vi "GV_YscaleAddText.vi"(4 "Color":u32(colorbox), 6 "X-position":i16, 7 "Tagname":string, 8 "Scale top":i16, 9 "Plot bottom":i16, 11 "2D Picture IN":picture) -> (3 "2D Picture OUT":picture)   [LabVIEW 2020, in "Sgraph_lib_V1.lvlib" / "Gviewer.lvclass"]
doc: "Andre Koelewijn, 25 July 2021\n\nThis vi will add a tagname to the Y scale."
uses:
  Gviewer.lvclass
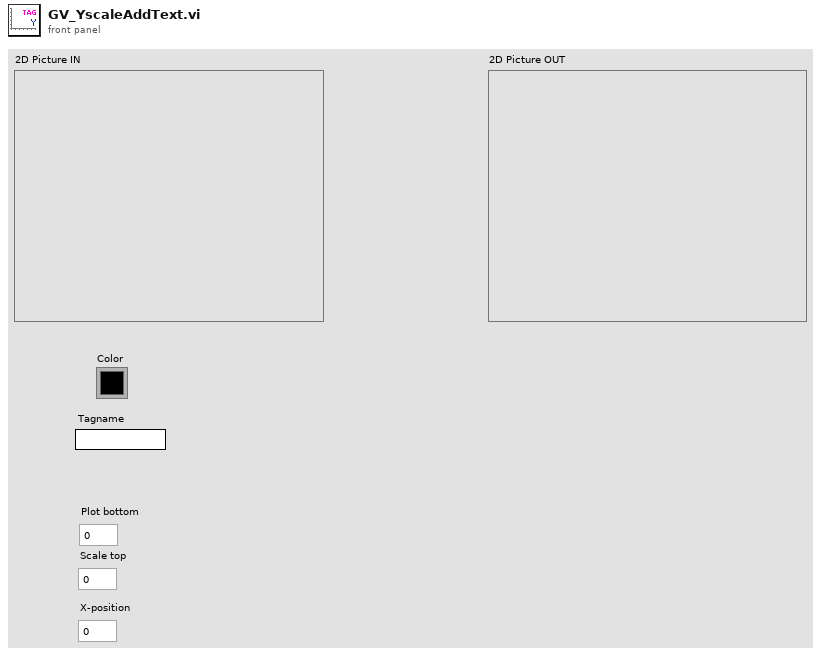
[diagram p1: front panel]
types:
  T1 = cluster{"horizontal":enum16{"left", "center", "right"}, "vertical":enum16{"top", "center", "bottom"}}
  T2 = cluster{"left":i16, "top":i16, "right":i16, "bottom":i16}
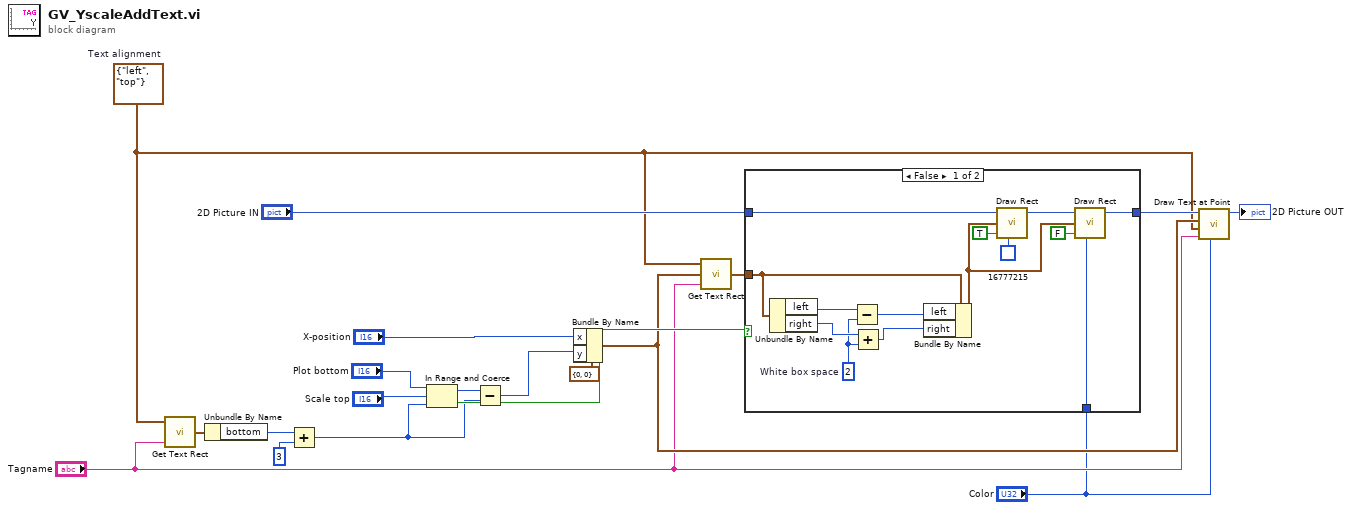
[diagram p0: block diagram]
diagram:
  w5 = T1 {"horizontal"=enum."left", "vertical"=enum."top"}  # Text alignment
  n1 = call <vilib>:"Get Text Rect.vi"("alignment(left, top)"=w5, "text"="Tagname") -> ("rect"=w13:T2)  [unwired: 7 in]
  n2 = Unbundle By Name(w13) -> ("bottom"=w12:i16)
  n3 = Add(x=w12, y=i16 3) -> (x+y=w2:i16)
  n4 = In Range and Coerce(upper limit="Plot bottom", x="Scale top", lower limit=w2) -> (coerced(x)=w10:i16, In Range?=w18:bool)
  n5 = Subtract(x=w10, y=w2) -> (x-y=w8:i16)
  n6 = Bundle By Name(cluster=cluster{"x":i16, "y":i16} {"x"=0, "y"=0} ("origin"), "x"="X-position", "y"=w8) -> (w7:cluster{"x":i16, "y":i16})
  n7 = call <vilib>:"Get Text Rect.vi"("alignment(left, top)"=w5, "origin(0,0)"=w7, "text"="Tagname") -> ("rect"=w4:T2)  [unwired: 6 in]
  n8 = case shown="False" w18 {
    tunnel: "2D Picture IN" -> [w33 w34]
    tunnel: [w31 w34] -> w16
    tunnel: w4 -> [w26 _]
    tunnel: "Color" -> [w29 _]
    frame False {
      w21 = i16 2  # White box space
      n9 = Unbundle By Name(w26) -> ("left"=w25:i16, "right"=w23:i16)
      n10 = Subtract(x=w25, y=w21) -> (x-y=w24:i16)
      n11 = Add(x=w23, y=w21) -> (x+y=w22:i16)
      n12 = Bundle By Name(cluster=w26, "left"=w24, "right"=w22) -> (w20:T2)
      n13 = call <vilib>:"Draw Rect.vi"("picture"=w33, "rect"=w20, "fill?(F)"=TRUE, "color(black)"=u32 16777215) -> ("new picture"=w32:picture)  [unwired: 5 in]
      n14 = call <vilib>:"Draw Rect.vi"("picture"=w32, "rect"=w20, "fill?(F)"=FALSE, "color(black)"=w29) -> ("new picture"=w31:picture)  [unwired: 5 in]
    }
    frame True {
    }
  }
  n15 = call <vilib>:"Draw Text at Point.vi"("text color(black)"="Color", "text"="Tagname", "alignment(left, top)"=w5, "origin"=w7, "picture"=w16) -> ("new picture"=→"2D Picture OUT":picture)  [unwired: 5 in, 1 out]
